vi "GetVisibleIncDec.vi"(8 "error in":errorcluster, 11 "SelList[]":refnum<vi>[](array[refnum])) -> (0 "error out":errorcluster, 3 "NumericRefs":refnum<vi>[](array[refnum]))   [LabVIEW 2016, in "Align Elements.lvlib"]
doc: "This VI will show or hide all Inc/Dec buttons in the selection. Errors won't make it out."
uses:
  Align Elements.lvlib
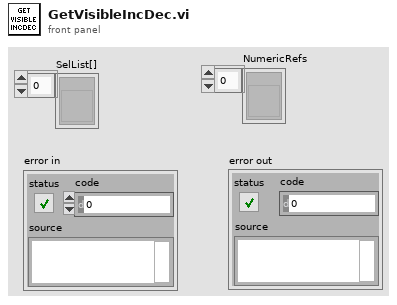
[diagram p1: front panel]
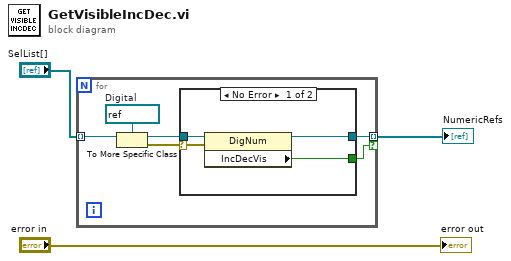
[diagram p0: block diagram]
diagram:
  n1 = for {
    tunnel: "SelList[]" -> [w9] mode=indexing
    tunnel: [w5] -> w1 mode=indexing if=w4
    w7 = refnum<vi> refnum  # Digital
    n2 = To More Specific Class(target class=w7, reference=w9) -> (specific class reference=w8:refnum<vi>, error out=w6:errorcluster)  [unwired: 1 in]
    n3 = case shown="No Error" w6 {
      selector: w6 -> [w13 _]
      tunnel: w8 -> [w12 w14]
      tunnel: [w11 w14] -> w5
      tunnel: [w10 _] -> w4
      frame No Error {
        n4 = property class="DigNum"(reference=w12, error in=w13) -> (reference out=w11:refnum<vi>, "IncDecVis"=w10:bool)  [unwired: 1 out]
      }
      frame Error {
      }
    }
  }
  "NumericRefs" <- w1
  "error out" <- "error in"
